vi "lab session 3.2.vi"() -> ()   [LabVIEW 2020]
panel:
  out "root 2":dbl
  out "root1":dbl
  in  "c":dbl
  in  "b":dbl
  in  "a":dbl
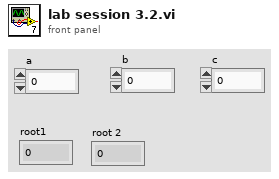
[diagram p1: front panel]
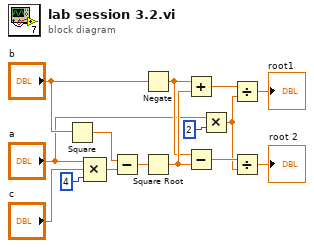
[diagram p0: block diagram]
diagram:
  n1 = Square(x="b") -> (x^2=w12:dbl)
  n2 = Compound Arithmetic op=MULTIPLY("a", "c", 4) -> (w11:dbl)
  n3 = Subtract(x=w12, y=w11) -> (x-y=w10:dbl)
  n4 = Negate(x="b") -> (-x=w8:dbl)
  n5 = Square Root(x=w10) -> (sqrt(x)=w9:dbl)
  n6 = Add(x=w8, y=w9) -> (x+y=w6:dbl)
  n7 = Subtract(x=w8, y=w9) -> (x-y=w5:dbl)
  n8 = Multiply(x="a", y=2) -> (x*y=w4:dbl)
  n9 = Divide(x=w6, y=w4) -> (x/y=→"root1":dbl)
  n10 = Divide(x=w5, y=w4) -> (x/y=→"root 2":dbl)
